vi "Tektronix 7000 Series Glitch Triggered Acquisition Waveform.vi"() -> ()   [LabVIEW 2015]
doc: "This example VI illustrates how to configure an oscilloscope to generate a glitch trigger and acquire a waveform from that trigger."
uses:
  <instrlib>/Tektronix 7000 Series/Public/Configure/Configure Trigger (A Mode).vi
  <instrlib>/Tektronix 7000 Series/Public/Configure/Configure Trigger (Glitch).vi
  <instrlib>/Tektronix 7000 Series/Public/Configure/Configure Trigger (Pattern).vi
  <instrlib>/Tektronix 7000 Series/Public/Data/Read (Single Waveform).vi
  <instrlib>/Tektronix 7000 Series/Tektronix 7000 Series.lvlib
panel:
  in  "Record Length (10000)":u32=10000 caption="Record Length (10000s)"
  in  "Channel4 Input":T1={"Channel4 Logical Input (0:High)"=0, "Channel4 Threshold (1.0v)  "=1.0} {"Channel4 Logical Input (0:High)" items=["High", "Low", "X"]}
  in  "Channel3 Input":T2={"Channel3 Logical Input (0:High)"=0, "Channel3 Threshold (1.0v)"=1.0} {"Channel3 Logical Input (0:High)" items=["High", "Low", "X"]}
  in  "Probe Attenuation (10.0)":dbl=10.0
  in  "Pattern Type (0:AND)":u16(ring) items=["AND", "NAND", "OR", "NOR"]
  in  "Time Holdoff (0.000001s)":dbl=1e-06
  in  "Holdoff Type (0:Auto)":u16(ring) items=["Auto", "Time", "Random", "Default"]
  in  "Trigger Mode (0:Normal)":u16(ring) items=["Normal", "Auto"]
  in  "Trigger Level (0)":dbl
  in  "Trigger if Glitch (0:Occurs)":u16(ring) items=["Occurs", "Logic"]
  in  "Timebase (0.005 s)":dbl=0.005
  in  "Channel (0: Channel 1)":u16(ring) format="%#_5f" items=["Channel 1", "Channel 2", "Channel 3", "Channel 4", "Math 1", "Math 2", "Math 3", "Math 4", "Reference 1", "Reference 2", "Reference 3", "Reference 4"]
  in  "Vertical Coupling (1: DC)":u16(ring)=1 items=["AC", "DC", "Ground"]
  in  "Vertical Range (10.0 V)":dbl=10.0
  out "Waveform Graph":waveform(dbl)(graph)
  in  "VISA Resource Name":refnum<visa-resource-name>
  # "(c) 2006 - 2016 National Instruments Corporation.  ALL RIGHTS RESERVED."
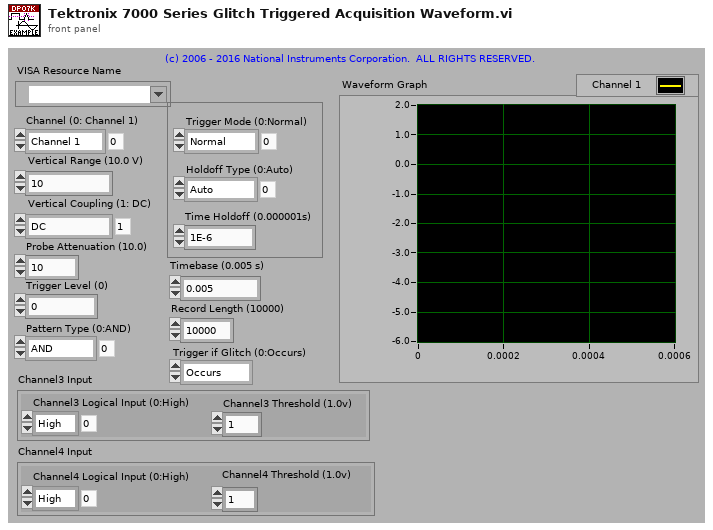
[diagram p1: front panel]
types:
  T1 = cluster{"Channel4 Logical Input (0:High)":u16, "Channel4 Threshold (1.0v)  ":dbl}
  T2 = cluster{"Channel3 Logical Input (0:High)":u16, "Channel3 Threshold (1.0v)":dbl}
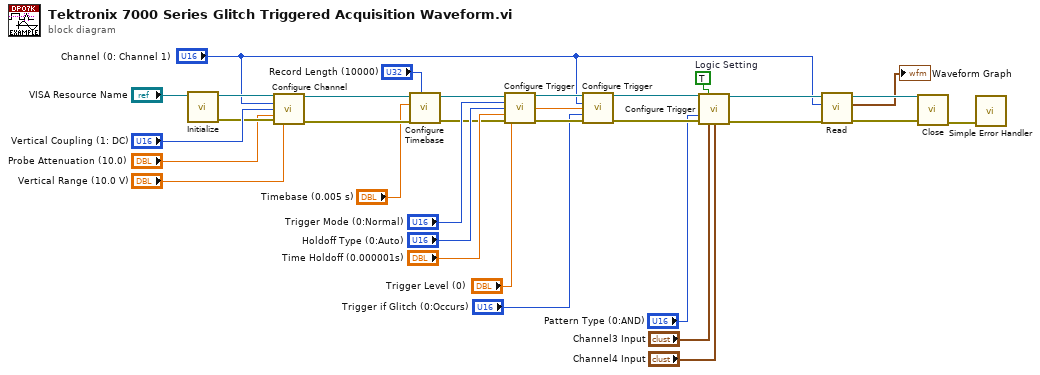
[diagram p0: block diagram]
diagram:
  w10 = TRUE  # Logic Setting
  n1 = call <instrlib>:"Initialize.vi"("VISA resource name"="VISA Resource Name") -> ("error out"=w12:errorcluster, "VISA resource name out"=w13:refnum<visa-resource-name>)  [unwired: 9 in]
  n2 = call <instrlib>:"Configure Channel.vi"("VISA resource name"=w13, "Channel (0: Channel 1)"="Channel (0: Channel 1)", "Vertical Coupling (1: DC)"="Vertical Coupling (1: DC)", "Probe Attenuation (1.0)"="Probe Attenuation (10.0)", "error in (no error)"=w12, "Vertical Range (10.0 V)"="Vertical Range (10.0 V)") -> ("VISA resource name out"=w15:refnum<visa-resource-name>, "error out"=w16:errorcluster)  [unwired: 8 in]
  n3 = call <instrlib>:"Configure Timebase.vi"("Record Length (10000)"="Record Length (10000)", "error in (no error)"=w16, "Timebase (4 ns)"="Timebase (0.005 s)", "VISA resource name"=w15) -> ("error out"=w8:errorcluster, "VISA resource name out"=w9:refnum<visa-resource-name>)  [unwired: 6 in]
  n4 = call-poly <instrlib>:"Configure Trigger.vi"("VISA resource name"=w9, "Trigger Mode (0:Normal)"="Trigger Mode (0:Normal)", "Holdoff Type (0:Auto)"="Holdoff Type (0:Auto)", "Time Holdoff (1us)"="Time Holdoff (0.000001s)", "error in (no error)"=w8) -> ("VISA resource name out"=w28:refnum<visa-resource-name>, "error out"=w27:errorcluster)  [unwired: 9 in]
  n5 = call-poly <instrlib>:"Configure Trigger.vi"("VISA resource name"=w28, "Source (0:Channel1)"="Channel (0: Channel 1)", "Trigger Level (0)"="Trigger Level (0)", "Trigger Condition (0:Less Than)"="Trigger if Glitch (0:Occurs)", "error in (no error)"=w27) -> ("VISA resource name out"=w25:refnum<visa-resource-name>, "error out"=w24:errorcluster)  [unwired: 8 in, 1 out]
  n6 = call-poly <instrlib>:"Configure Trigger.vi"("VISA resource name"=w25, "Logic Setting (False)"=w10, "Pattern Type (0:AND)"="Pattern Type (0:AND)", "error in (no error)"=w24, "Channel3 Input"="Channel3 Input", "Channel4 Input"="Channel4 Input") -> ("VISA resource name out"=w23:refnum<visa-resource-name>, "error out"=w22:errorcluster)  [unwired: 8 in]
  n7 = call-poly <instrlib>:"Read.vi"("error in (no error)"=w22, "Channel (0: Channel 1)"="Channel (0: Channel 1)", "VISA resource name"=w23) -> ("error out"=w5:errorcluster, "Waveform Data"=→"Waveform Graph":waveform(dbl), "VISA resource name out"=w20:refnum<visa-resource-name>)  [unwired: 6 in]
  n8 = call <instrlib>:"Close.vi"("error in (no error)"=w5, "VISA resource name"=w20) -> ("error out"=w21:errorcluster)  [unwired: 9 in]
  n9 = call <vilib>:"Simple Error Handler.vi"("error in (no error)"=w21) -> ()  [unwired: 4 in, 5 out]
